vi "HandleExit.vi"(8 "error in (no error)":errorcluster, 9 "VI Refnum":refnum<vi>, 10 "StopArgument":variant, 11 "ModuleAdmin":refnum<class "ModuleAdmin.lvclass">) -> (0 "error out":errorcluster, 1 "Exit via Stop Module Req?":bool, 2 "WaitForStop?":bool)   [LabVIEW 2018, in "MyPlugins.lvlib"]
doc: "Sends a message to stop the clone."
uses:
  MyPlugins.lvlib
  <userlib>/NIST/ModuleAdminLib/ModuleAdmin/ModuleAdmin.lvclass
  C:/Program Files (x86)/National Instruments/LabVIEW 2018/user.lib/NIST/ModuleAdminLib/ModuleAdminBase/ModuleAdminBase.lvclass
  PluginsShared/clStopArgument.ctl
  PluginsShared/PluginsShared.lvlib
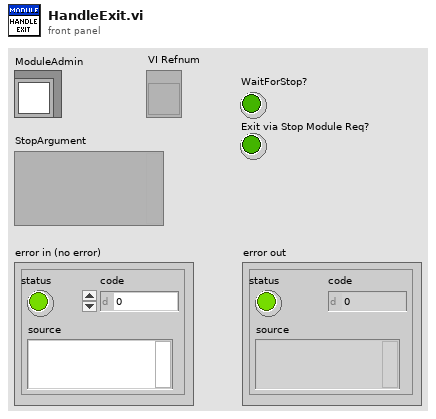
[diagram p1: front panel]
types:
  T1 = typedef "PluginsShared.lvlib/clStopArgument.ctl" = cluster{"Exit via Stop Module Req?":bool, "Wait for Module to stop?":bool, "ModuleAdmin":refnum<class "ModuleAdmin.lvclass">}
  T2 = enum32{"Invalid", "Standard", "Closed", "Hidden", "Minimized", "Maximized"}
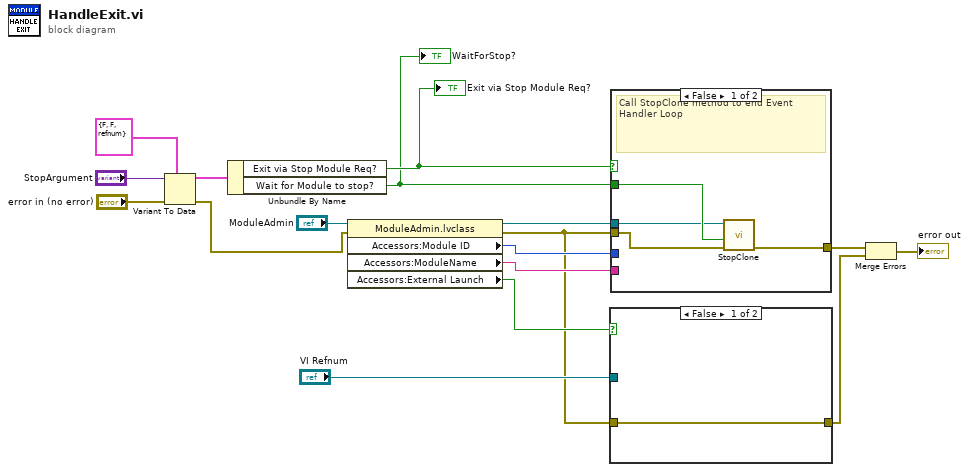
[diagram p0: block diagram]
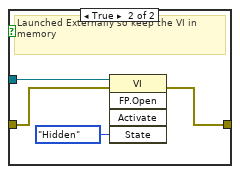
[diagram p2: hidden frame]
diagram:
  n1 = Variant To Data(error in="error in (no error)", type=T1 {"Exit via Stop Module Req?"=FALSE, "Wait for Module to stop?"=FALSE, "ModuleAdmin"=refnum} ("Stop Argument"), Variant="StopArgument") -> (data=w12:T1, error out=w3:errorcluster)
  n2 = Unbundle By Name(w12) -> ("Exit via Stop Module Req?"=w7:bool, "Wait for Module to stop?"=w5:bool)
  "WaitForStop?" <- w5
  "Exit via Stop Module Req?" <- w7
  n3 = property class="ModuleAdmin.lvclass"(reference="ModuleAdmin", error in=w3) -> (reference out=w4:refnum<class "ModuleAdmin.lvclass">, error out=w1:errorcluster, "Accessors:Module ID"=w8:i32, "Accessors:ModuleName"=w9:string, "Accessors:External Launch"=w10:bool)
  n4 = case shown="False" w10 {
    tunnel: "VI Refnum" -> [_ w22]
    tunnel: [w18 w20] -> w15
    tunnel: w1 -> [w18 w19]
    frame False {
    }
    frame True {
      # "Launched Externally so keep the VI in memory"
      n5 = invoke class="VI" method="FP.Open"(reference=w22, error in=w19, "State"=T2."Hidden") -> (error out=w20:errorcluster)  [unwired: 2 in, 4 out]
    }
  }
  n6 = case shown="False" w7 {
    tunnel: w8 -> [_ _]
    tunnel: [w26 _] -> w16
    tunnel: w9 -> [_ _]
    tunnel: w5 -> [w25 _]
    tunnel: w4 -> [w24 _]
    tunnel: w1 -> [w23 _]
    frame False {
      # "Call StopClone method to end Event Handler Loop"
      n7 = call "StopClone.vi"("error in (no error)"=w23, "Wait for Module to stop?"=w25, "ModuleAdmin"=w24) -> ("error out"=w26:errorcluster)  [unwired: 8 in]
    }
    frame True {
      # "This came from the Event Handler Loop"
    }
  }
  n8 = Merge Errors(w16, w15) -> (→"error out":errorcluster)
